vi "Find Peak Attributes V2.vi"(0 "Intensity Data":dbl[](array[numeric]), 1 "Threshold":dbl format="%0.2f", 2 "Pixel Saturation":dbl=225.0, 3 "error in (no error)":errorcluster) -> (4 "XY Intensity Plot":cluster{i32[], "Best Gaussian Fit":dbl[]}[](array[cluster]), 5 "peak location":dbl, 6 "peak amplitude":dbl, 7 "peak width":dbl, 8 "error out":errorcluster)   [LabVIEW 2012]
uses:
  <vilib>/Analysis/NI_AAL_SigProc.lvlib
  <vilib>/Analysis/NI_AALPro.lvlib
panel:
  out "amplitude":dbl
  out "test plot":cluster{i32[], "Best Gaussian Fit":dbl[]}[](graph)
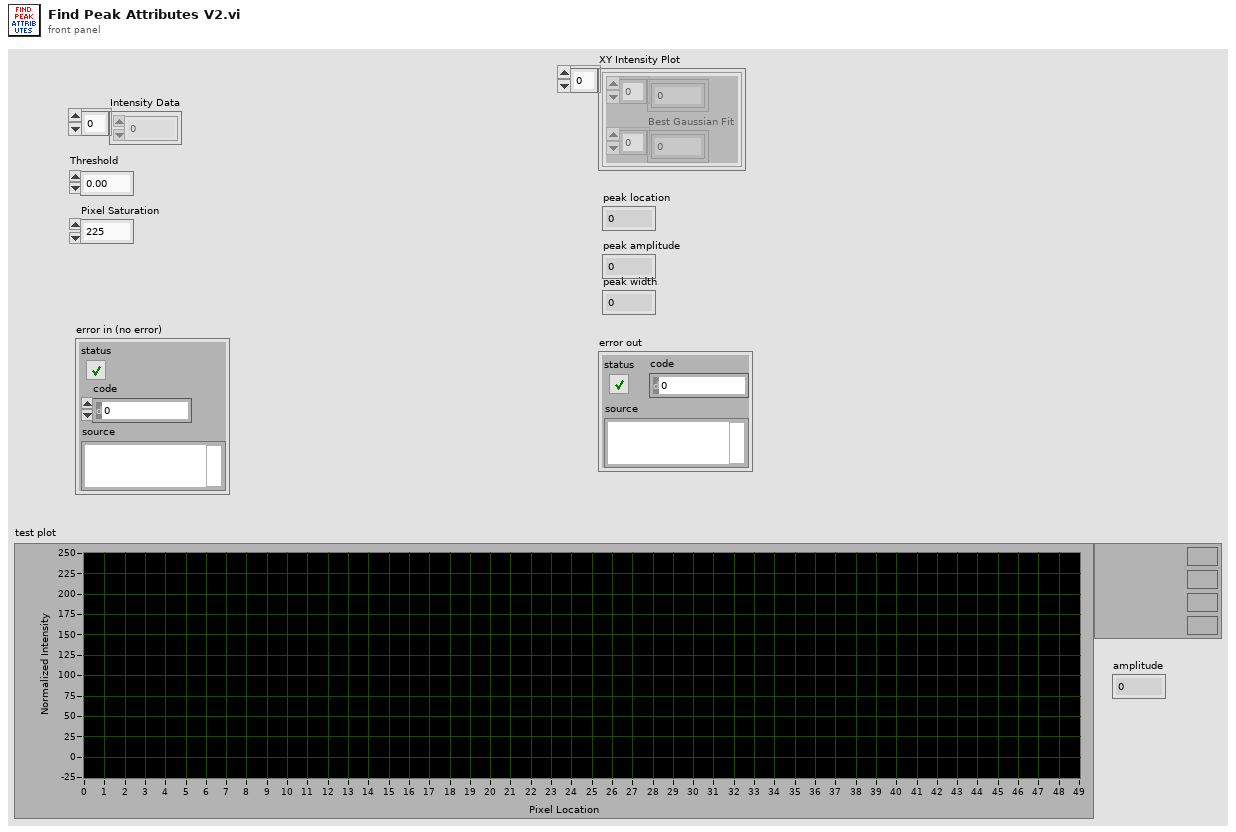
[diagram p1: front panel]
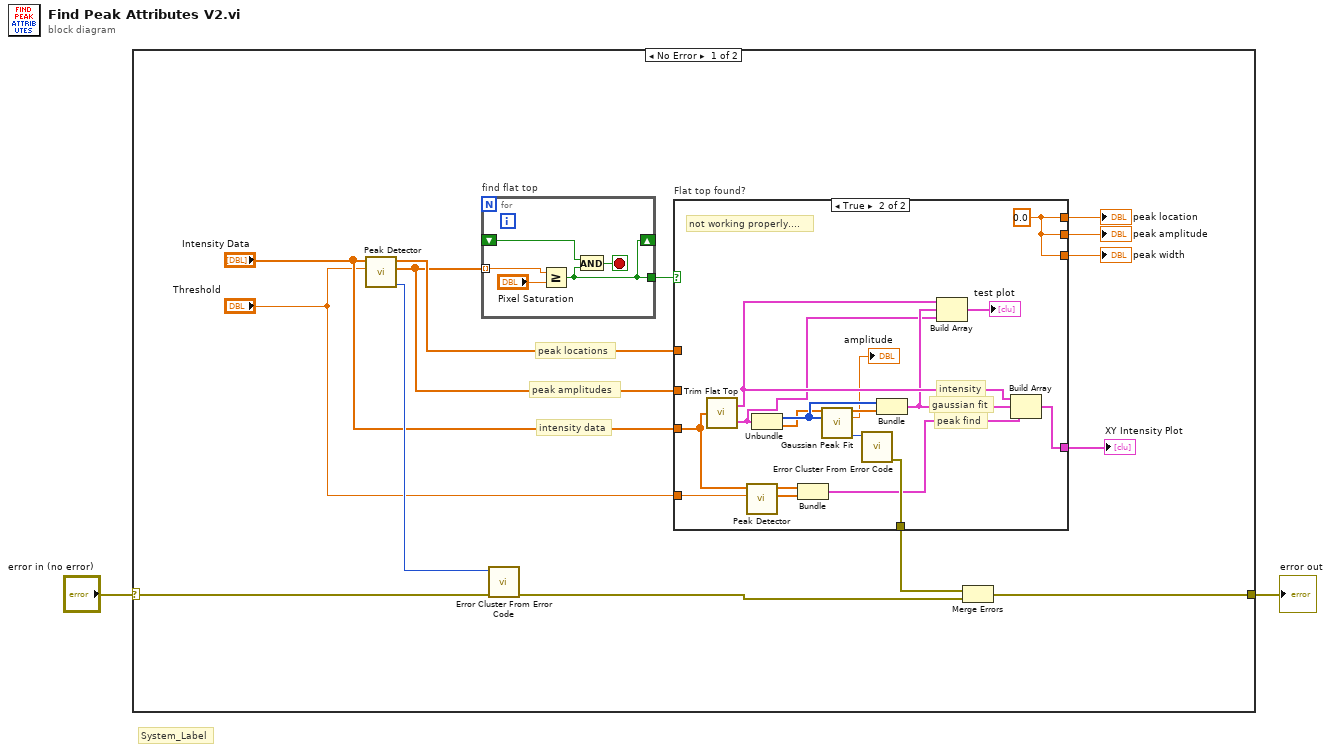
[diagram p0: block diagram]
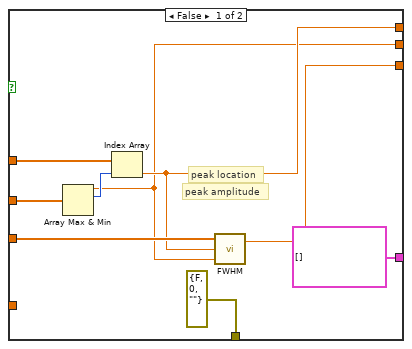
[diagram p2: hidden frame]
diagram:
  # "System_Label"
  n1 = case shown="No Error" "error in (no error)" {
    selector: "error in (no error)" -> [w11 w48]
    tunnel: [w4 w48] -> w1
    frame No Error {
      # "intensity data"
      # "peak amplitudes"
      # "peak locations"
      n2 = call <vilib>:"Peak Detector.vi"("threshold"="Threshold", "X"="Intensity Data") -> ("error"=w16:i32, "Amplitudes"=w13:dbl[], "Locations"=w14:dbl[])  [unwired: 5 in, 2 out]
      n3 = for "find flat top" {
        tunnel: w13 -> [w46] mode=indexing
        tunnel: [w43] -> w15
        shift-right: [w43] -> _
        shift-left: _ -> [w44]
        stop <- w45 stop-if-true
        n4 = Greater Or Equal?(x=w46, y="Pixel Saturation") -> (x >= y?=w43:bool)
        n5 = And(x=w44, y=w43) -> (x .and. y?=w45:bool)
      }
      n6 = call <vilib>:"Error Cluster From Error Code.vi"("error in (no error)"=w11, "error code (0)"=w16) -> ("error out"=w5:errorcluster)  [unwired: 7 in]
      n7 = case "Flat top found?" shown="True" w15 {
        tunnel: w14 -> [w23 _]
        tunnel: w13 -> [w25 _]
        tunnel: [w20 w42] -> w9
        tunnel: [w21 w42] -> w10
        tunnel: "Intensity Data" -> [w22 w35]
        tunnel: [w19 w42] -> w8
        tunnel: [cluster{i32[], "Best Gaussian Fit":dbl[]}[] [] w37] -> w7
        tunnel: [errorcluster {"status"=FALSE, "code"=0, "source"=""} ("error out") w36] -> w6
        tunnel: "Threshold" -> [_ w34]
        frame False {
          # "peak amplitude"
          # "peak location"
          n8 = Array Max & Min(array=w25) -> (max value=w20:dbl, max index (indices)=w24:i32)  [unwired: 2 out]
          n9 = Index Array(array=w23, index=w24) -> (element=w21:dbl)
          n10 = call "FWHM.vi"("Peak Amplitude"=w20, "Peak Location"=w21, "Intensity Data"=w22) -> ("Width"=w19:dbl)  [unwired: 1 out]
        }
        frame True {
          w42 = 0.0
          # "not working properly...."
          # "peak find"
          # "gaussian fit"
          # "intensity"
          n11 = call "Trim Flat Top.vi"("Data In"=w35) -> ("Data Out (x,y)"=w30:cluster{i32[], dbl[]}, "Trimmed Data (x,y)"=w26:cluster{i32[], dbl[]})
          n12 = call <vilib>:"Peak Detector.vi"("threshold"=w34, "X"=w35) -> ("Amplitudes"=w32:dbl[], "Locations"=w33:dbl[])  [unwired: 5 in, 3 out]
          n13 = Unbundle(w26) -> (w41:i32[], w40:dbl[])
          n14 = Bundle("Locations"=w33, "Amplitudes"=w32) -> (w31:cluster{"Locations":dbl[], "Amplitudes":dbl[]})  [unwired: 1 in]
          n15 = call <vilib>:"Gaussian Peak Fit.vi"("Y"=w40, "X"=w41) -> ("Best Gaussian Fit"=w38:dbl[], "amplitude"=→"amplitude":dbl, "error"=w39:i32)  [unwired: 7 in, 4 out]
          n16 = call <vilib>:"Error Cluster From Error Code.vi"("error code (0)"=w39) -> ("error out"=w36:errorcluster)  [unwired: 8 in]
          n17 = Bundle(w41, "Best Gaussian Fit"=w38) -> (w27:cluster{i32[], "Best Gaussian Fit":dbl[]})  [unwired: 1 in]
          n18 = Build Array(w30, w27, w26) -> (→"test plot":cluster{i32[], "Best Gaussian Fit":dbl[]}[])
          n19 = Build Array(w30, w27, w31) -> (w37:cluster{"Locations":dbl[], "Amplitudes":dbl[]}[])
        }
      }
      "peak location" <- w10
      "peak amplitude" <- w9
      "peak width" <- w8
      "XY Intensity Plot" <- w7
      n20 = Merge Errors(w6, w5) -> (w4:errorcluster)
    }
    frame Error {
    }
  }
  "error out" <- w1
